vi "1_Waveform_Signal_Classification(Training).vi"() -> ()   [LabVIEW 2020]
uses:
  <vilib>/Ngene/Deep Learning Toolkit/Toolkit/NN_Train/Controls/NN_LR_Policy_Cfg.ctl
  <vilib>/Ngene/Deep Learning Toolkit/Toolkit/NN_Train/Controls/NN_LR_Policy_Type.ctl
  <vilib>/Ngene/Deep Learning Toolkit/Toolkit/NN_Train/Controls/NN_Train_Session_Data.ctl
  <vilib>/Ngene/Deep Learning Toolkit/Toolkit/NN_Train/Controls/NN_Train_Params.ctl
  <vilib>/Ngene/Deep Learning Toolkit/Toolkit/NN_Train/Controls/NN_Train_Optimizer.ctl
  <vilib>/Ngene/Deep Learning Toolkit/Toolkit/NN_Train/Controls/NN_Train_Data_Sampling.ctl
  <vilib>/Ngene/Deep Learning Toolkit/Toolkit/NN_Network/Controls/NN_Device.ctl
  <vilib>/Ngene/Deep Learning Toolkit/Toolkit/NN_Train/Eval_Loss/NN_Eval_Test_Error_Loss/Controls/NN_Eval_Params.ctl
  <vilib>/Ngene/Deep Learning Toolkit/Toolkit/NN_Layers/Layers/Input/Controls/NN_Layer_Config(Input1D).ctl
  <vilib>/Ngene/Deep Learning Toolkit/Toolkit/NN_Data/Controls/NN_Data_type.ctl
  <vilib>/Ngene/Deep Learning Toolkit/Toolkit/NN_Layers/Layers/FC/Controls/NN_Layer_Config(FC).ctl
  <vilib>/Ngene/Deep Learning Toolkit/Toolkit/NN_Layers/Layers/BatchNorm/Controls/NN_BN_Params.ctl
  <vilib>/Ngene/Deep Learning Toolkit/Toolkit/NN_Activations/Controls/NN_Activation_Type.ctl
  <vilib>/Ngene/Deep Learning Toolkit/Toolkit/NN_Layers/Controls/NN_Layer_Init_Params.ctl
  <vilib>/Ngene/Deep Learning Toolkit/Toolkit/NN_Layers/Controls/NN_Layer_Weight_Init_Type.ctl
  <vilib>/Ngene/Deep Learning Toolkit/Toolkit/NN_Network/Controls/NN_Save_Before_Destroy_Options.ctl
  <vilib>/Ngene/Deep Learning Toolkit/Toolkit/NN_Layers/Layers/Input/NN_Layer_Create(Input1D).vi
  <vilib>/Ngene/Deep Learning Toolkit/Toolkit/NN_Layers/Layers/FC/NN_Layer_Create(FC).vi
  <vilib>/Ngene/Deep Learning Toolkit/Toolkit/NN_Layers/Layers/SoftMax/NN_Layer_Create(SoftMax).vi
  <vilib>/Ngene/Deep Learning Toolkit/Toolkit/NN_Train/Loss_Functions/NN_Set_Loss(CrossEntropy).vi
  <vilib>/Ngene/Deep Learning Toolkit/Toolkit/NN_Network/subVIs/NN_Predict/NN_Predict(In1D_Out1D).vi
  <vilib>/Ngene/Deep Learning Toolkit/Toolkit/NN_Train/Eval_Loss/NN_Eval_Test_Error_Loss/NN_Eval(In1D_Out1D).vi
  <vilib>/Ngene/Deep Learning Toolkit/Toolkit/Deep_Learning_Toolkit_by_Ngene.lvlib
  <vilib>/ptbypt/NI_PtbyPt.lvlib
panel:
  out "Eval_Results":T1
  out "Training Loss":sgl=0.03360607 format="%#.6g"
  in  "Eval":bool
  out "Loss Graphs":cluster{"mean":dbl, "Loss":sgl}(graph)
  in  "NN_Device":T2
  in  "Stop Training":bool
  in  "NN_Train_Params":T3={"Optimizer"=enum."SGD", "Beta_1"=0.9, "Beta_2"=0.999, "Weight Decay(L1)"=1e-07, "Weight Decay(L2)"=1e-07, "Data_Sampling"=enum."Random"}
  out "Session Data":T6={"Epochs"=46.08768, "Tot_Iter"=36006, "LR"=3.90625e-05, "LR_iter"=36007}
  in  "LR Update Policy":T7={"Policy_Type"=enum."Step", "LR0"=0.02, "k"=5.0, "WarmUp_Policy"=enum."Ramp", "WarmUp_Iter"=100, "WarmUp_Ratio"=10.0} {"WarmUp_Ratio" min=1; "WarmUp_Iter" min=1; "LR0" format="%.7f"}
  # "Overview: This example demonstrating the usage of Deep Learning Toolkit for solving  waveform signal classification problem.\nRequirements: Deep Learning Toolkit for LabVIEW\nInstructions:\n1.  Run the VI with current configuration of the training parameters and Learning Rate update policy\n2. Observe how the training loss is decreasing\n3. Press the \"Stop Training\" when the loss is not decreasing any more."
  # "Waveform Signal Classifier - Training"
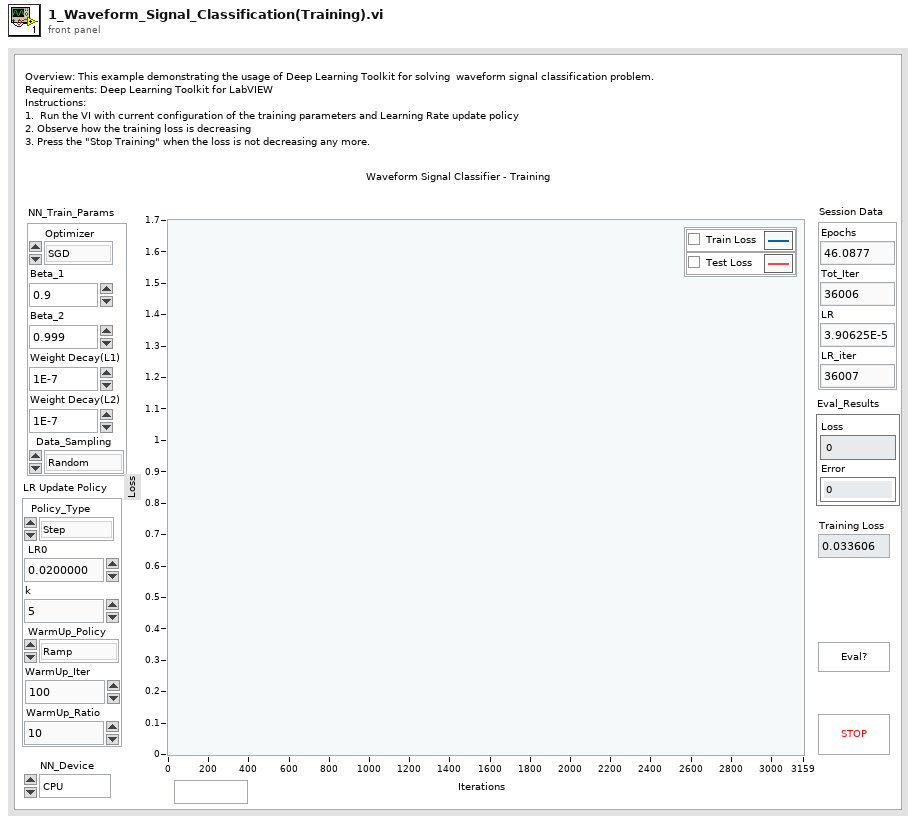
[diagram p1: front panel]
types:
  T1 = typedef "Deep_Learning_Toolkit_by_Ngene.lvlib/NN_Eval_Params.ctl" = cluster{"Loss":sgl, "Error":sgl}
  T2 = typedef "Deep_Learning_Toolkit_by_Ngene.lvlib/NN_Device.ctl" = enum16{"CPU", "GPU"}
  T3 = typedef "Deep_Learning_Toolkit_by_Ngene.lvlib/NN_Train_Params.ctl" = cluster{"Optimizer":T4, "Beta_1":sgl, "Beta_2":sgl, "Weight Decay(L1)":sgl, "Weight Decay(L2)":sgl, "Data_Sampling":T5}
  T4 = typedef "Deep_Learning_Toolkit_by_Ngene.lvlib/NN_Train_Optimizer.ctl" = enum16{"SGD", "Adam", "Adagrad", "Adadelta", "RMSProp", "Nesterov"}
  T5 = typedef "Deep_Learning_Toolkit_by_Ngene.lvlib/NN_Train_Data_Sampling.ctl" = enum16{"Random", "Sequential"}
  T6 = typedef "Deep_Learning_Toolkit_by_Ngene.lvlib/NN_Train_Session_Data.ctl" = cluster{"Epochs":sgl, "Tot_Iter":i32, "LR":sgl, "LR_iter":i32}
  T7 = typedef "Deep_Learning_Toolkit_by_Ngene.lvlib/NN_LR_Policy_Cfg.ctl" = cluster{"Policy_Type":T8, "LR0":dbl, "k":sgl, "WarmUp_Policy":enum16{"Step", "Ramp"}, "WarmUp_Iter":i32, "WarmUp_Ratio":sgl}
  T8 = typedef "Deep_Learning_Toolkit_by_Ngene.lvlib/NN_LR_Policy_Type.ctl" = enum16{"Manual", "Step", "Exp", "1/t"}
  T9 = typedef "Deep_Learning_Toolkit_by_Ngene.lvlib/NN_Save_Before_Destroy_Options.ctl" = cluster{"CFG?":bool, "Weights?":bool, "Render?":bool}
  T10 = typedef "Deep_Learning_Toolkit_by_Ngene.lvlib/NN_Layer_Config(FC).ctl" = cluster{"Name":string, "Size":i32, "BN":bool, "BN_Params":T11, "Activation":T12, "Has Bias?":bool, "Init_Params":T13, "Custom_Params":string}
  T11 = typedef "Deep_Learning_Toolkit_by_Ngene.lvlib/NN_BN_Params.ctl" = cluster{"epsilon":sgl, "momentum":sgl}
  T12 = typedef "Deep_Learning_Toolkit_by_Ngene.lvlib/NN_Activation_Type.ctl" = enum16{"Sigmoid", "ReLU", "LReLU", "ReLU6", "GELU", "tanh", "Swish", "Mish", "None"}
  T13 = typedef "Deep_Learning_Toolkit_by_Ngene.lvlib/NN_Layer_Init_Params.ctl" = cluster{"Init_Type":T14, "Value":sgl}
  T14 = typedef "Deep_Learning_Toolkit_by_Ngene.lvlib/NN_Layer_Weight_Init_Type.ctl" = enum16{"Const", "Uniform", "Gaussian", "Xavier"}
  T15 = typedef "Deep_Learning_Toolkit_by_Ngene.lvlib/NN_Layer_Config(Input1D).ctl" = cluster{"Name":string, "Size":i32, "Data_Type":T16, "Shift":sgl, "Scale":sgl}
  T16 = typedef "Deep_Learning_Toolkit_by_Ngene.lvlib/NN_Data_type.ctl" = enum16{"I8", "U8", "I16", "U16", "U32 ARGB", "SGL"}
  T17 = typedef "Deep_Learning_Toolkit_by_Ngene.lvlib/NN_DataSets_All(In1D_Out1D).ctl" = cluster{"Train":T18, "Validation":T18, "Test":T18}
  T18 = typedef "Deep_Learning_Toolkit_by_Ngene.lvlib/NN_DataSet(In1D_Out1D).ctl" = cluster{"Inputs Ref.":variant, "Outputs Ref.":T19, "Dims_In":i32, "Dataset_Size":i32, "Dims_Out":i32, "Labels":string[], "File Paths":path[], "Custom_Data":variant}
  T19 = typedef "Deep_Learning_Toolkit_by_Ngene.lvlib/NN_Data_ref(2D_SGL).ctl" = refnum<data-value>
  T20 = typedef "Deep_Learning_Toolkit_by_Ngene.lvlib/NN.ctl" = cluster{"Name":string, "No of Layers":i32, "mBatch":i32, "Layers":T21[], "Dimty":T22, "Dims_In":T23, "Dims_Out":T23, "Working_Dir":path, "Train?":bool, "Train_Params":T3, "LR_Update_Policy":T7, "Session Data":T6, "Ground_truth":T24, "NNg_hdls":T25, "NN_Device":T2, "GPU Id":i32, "Labels":string[], "Loss_Type":T26, "Loss_Cfg_Prms":variant, "NNG_WS":T27, "DryRun?":bool}
  T21 = typedef "Deep_Learning_Toolkit_by_Ngene.lvlib/NN_Layer_ref.ctl" = refnum<file>
  T22 = typedef "Deep_Learning_Toolkit_by_Ngene.lvlib/NN_In_Out_Dim-ty.ctl" = enum8{"In1D_Out1D", "In3D_Out1D", "In3D_Out3D", "In3D_OutBBox"}
  T23 = typedef "Deep_Learning_Toolkit_by_Ngene.lvlib/NN_Dims(C,H,W).ctl" = cluster{"C":i32, "H":i32, "W":i32}
  T24 = typedef "Deep_Learning_Toolkit_by_Ngene.lvlib/NN_Ground_truth.ctl" = cluster{"Y":variant}
  T25 = typedef "Deep_Learning_Toolkit_by_Ngene.lvlib/nng_cuda_handles.ctl" = cluster{"cudnn":u64, "cublas":u64, "stream":u64, "curand":u64}
  T26 = typedef "Deep_Learning_Toolkit_by_Ngene.lvlib/NN_Loss_Type.ctl" = enum16{"None", "MSE", "CrossEntropy", "YOLO_v2", "YOLO_v4"}
  T27 = typedef "Deep_Learning_Toolkit_by_Ngene.lvlib/NNG_WS.ctl" = cluster{"NNG_WS_Mem":T28, "Max_WS_Size":i64}
  T28 = typedef "Deep_Learning_Toolkit_by_Ngene.lvlib/NNg_WS_Mem_DVR.ctl" = refnum<data-value>
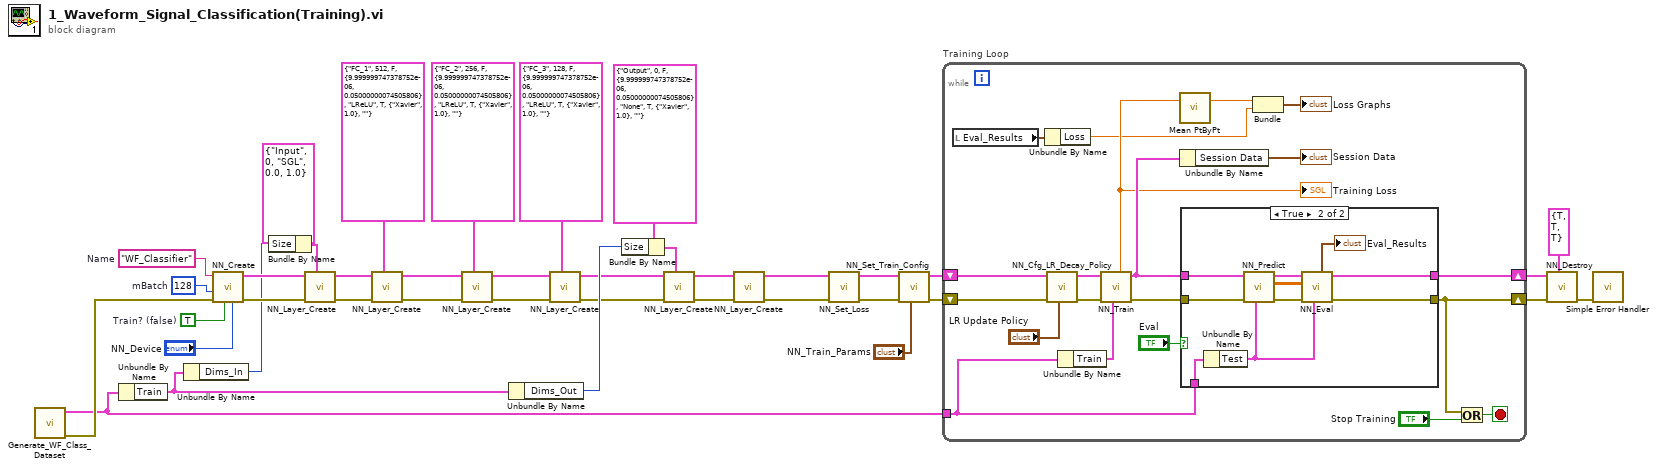
[diagram p0: block diagram]
diagram:
  w18 = "WF_Classifier"  # Name
  w19 = 128  # mBatch
  w20 = TRUE  # Train? (false)
  n1 = call "Generate_WF_Class_Dataset.vi"() -> ("error out"=w30:errorcluster, "DataSets_All(In1D_Out1D)"=w2:T17)  [unwired: 10 in]
  n2 = Unbundle By Name(w2) -> ("Train"=w23:T18)
  n3 = Unbundle By Name(w23) -> ("Dims_In"=w28:i32)
  n4 = call <vilib>:"NN_Create.vi"("NN_Device"="NN_Device", "Train? (false)"=w20, "error in (no error)"=w30, "mBatch (1)"=w19, "Name"=w18) -> ("error out"=w38:errorcluster, "NN out"=w39:T20)  [unwired: 5 in]
  n5 = Bundle By Name(cluster=T15 {"Name"="Input", "Size"=0, "Data_Type"=enum."SGL", "Shift"=0.0, "Scale"=1.0} ("Input1D_Cfg"), "Size"=w28) -> (w29:T15)
  n6 = call-poly <vilib>:"NN_Layer_Create.vi"("Input1D_Cfg"=w29, "error in (no error)"=w38, "NN in"=w39) -> ("error out"=w24:errorcluster, "NN out"=w25:T20)  [unwired: 6 in, 1 out]
  n7 = call-poly <vilib>:"NN_Layer_Create.vi"("FC_Cfg"=T10 {"Name"="FC_1", "Size"=512, "BN"=FALSE, "BN_Params"={"epsilon"=1e-05, "momentum"=0.05}, "Activation"=enum."LReLU", "Has Bias?"=TRUE, "Init_Params"={"Init_Type"=enum."Xavier", "Value"=1.0}, "Custom_Params"=""} ("FC_Cfg_1"), "error in (no error)"=w24, "NN in"=w25) -> ("error out"=w11:errorcluster, "NN out"=w12:T20)  [unwired: 6 in, 1 out]
  n8 = call-poly <vilib>:"NN_Layer_Create.vi"("FC_Cfg"=T10 {"Name"="FC_2", "Size"=256, "BN"=FALSE, "BN_Params"={"epsilon"=1e-05, "momentum"=0.05}, "Activation"=enum."LReLU", "Has Bias?"=TRUE, "Init_Params"={"Init_Type"=enum."Xavier", "Value"=1.0}, "Custom_Params"=""} ("FC_Cfg_1"), "error in (no error)"=w11, "NN in"=w12) -> ("error out"=w7:errorcluster, "NN out"=w8:T20)  [unwired: 6 in, 1 out]
  n9 = Unbundle By Name(w23) -> ("Dims_Out"=w26:i32)
  n10 = call-poly <vilib>:"NN_Layer_Create.vi"("FC_Cfg"=T10 {"Name"="FC_3", "Size"=128, "BN"=FALSE, "BN_Params"={"epsilon"=1e-05, "momentum"=0.05}, "Activation"=enum."LReLU", "Has Bias?"=TRUE, "Init_Params"={"Init_Type"=enum."Xavier", "Value"=1.0}, "Custom_Params"=""} ("FC_Cfg_1"), "error in (no error)"=w7, "NN in"=w8) -> ("error out"=w5:errorcluster, "NN out"=w6:T20)  [unwired: 6 in, 1 out]
  n11 = Bundle By Name(cluster=T10 {"Name"="Output", "Size"=0, "BN"=FALSE, "BN_Params"={"epsilon"=1e-05, "momentum"=0.05}, "Activation"=enum."None", "Has Bias?"=TRUE, "Init_Params"={"Init_Type"=enum."Xavier", "Value"=1.0}, "Custom_Params"=""} ("FC_Cfg_1"), "Size"=w26) -> (w27:T10)
  n12 = call-poly <vilib>:"NN_Layer_Create.vi"("FC_Cfg"=w27, "error in (no error)"=w5, "NN in"=w6) -> ("error out"=w33:errorcluster, "NN out"=w34:T20)  [unwired: 6 in, 1 out]
  n13 = call-poly <vilib>:"NN_Layer_Create.vi"("error in (no error)"=w33, "NN in"=w34) -> ("error out"=w15:errorcluster, "NN out"=w35:T20)  [unwired: 7 in, 1 out]
  n14 = call-poly <vilib>:"NN_Set_Loss.vi"("error in (no error)"=w15, "NN in"=w35) -> ("error out"=w14:errorcluster, "NN out"=w16:T20)  [unwired: 8 in]
  n15 = call <vilib>:"NN_Set_Train_Config.vi"("NN_Train_Params"="NN_Train_Params", "error in (no error)"=w14, "NN in"=w16) -> ("error out"=w21:errorcluster, "NN out"=w22:T20)  [unwired: 7 in]
  n16 = while "Training Loop" {
    shift-right: [w45] -> w3
    shift-left: w21 -> [w54]
    shift-right: [w50] -> w4
    shift-left: w22 -> [w57]
    tunnel: w2 -> [w43]
    stop <- w46 stop-if-true
    n17 = local read "Eval_Results"() -> (w41:T1)
    n18 = Unbundle By Name(w41) -> ("Loss"=w40:sgl)
    n19 = call <vilib>:"NN_Cfg_LR_Decay_Policy.vi"("LR_Decay_Params"="LR Update Policy", "error in (no error)"=w54, "NN in"=w57) -> ("error out"=w55:errorcluster, "NN out"=w56:T20)  [unwired: 7 in]
    n20 = Unbundle By Name(w43) -> ("Train"=w42:T18)
    n21 = call <vilib>:"NN_Train.vi"("Train Dataset"=w42, "error in (no error)"=w55, "NN in"=w56) -> ("error out"=w51:errorcluster, "NN out"=w52:T20, "Loss"=w47:sgl)  [unwired: 3 in, 3 out]
    "Training Loss" <- w47
    n22 = call <vilib>:"Mean PtByPt.vi"("x"=w47) -> ("mean"=w44:dbl)  [unwired: 3 in, 1 out]
    n23 = Unbundle By Name(w52) -> ("Session Data"=→"Session Data":T6)
    n24 = case shown="True" "Eval" {
      tunnel: w52 -> [w61 w70]
      tunnel: w51 -> [w60 w69]
      tunnel: [w61 w68] -> w50
      tunnel: [w60 w65] -> w45
      tunnel: w43 -> [_ w64]
      frame False {
      }
      frame True {
        n25 = Unbundle By Name(w64) -> ("Test"=w63:T18)
        n26 = call-poly <vilib>:"NN_Predict.vi"("Dataset"=w63, "error in (no error)"=w69, "NN in"=w70) -> ("error out"=w71:errorcluster, "Predictions"=w66:sgl[][], "NN out"=w67:T20)  [unwired: 6 in]
        n27 = call-poly <vilib>:"NN_Eval.vi"("Dataset"=w63, "error in (no error)"=w71, "Predictions"=w66, "NN in"=w67) -> ("error out"=w65:errorcluster, "NN out"=w68:T20, "NN_Eval_Params"=→"Eval_Results":T1)  [unwired: 4 in, 1 out]
      }
    }
    n28 = Bundle("mean"=w44, "Loss"=w40) -> (→"Loss Graphs":cluster{"mean":dbl, "Loss":sgl})  [unwired: 1 in]
    n29 = Or(x=w45, y="Stop Training") -> (x .or. y?=w46:bool)
  }
  n30 = call <vilib>:"NN_Destroy.vi"("Save (T, T, T)"=T9 {"CFG?"=TRUE, "Weights?"=TRUE, "Render?"=TRUE}, "error in (no error)"=w3, "NN in"=w4) -> ("error out"=w32:errorcluster)  [unwired: 7 in, 1 out]
  n31 = call <vilib>:"Simple Error Handler.vi"("error in (no error)"=w32) -> ()  [unwired: 4 in, 5 out]
